vi "Name Strings to Version.vi"(9 "target name":string, 11 "robot model name (plugin name)":string) -> (0 "invalid inputs?":bool, 1 "FPGA target":T1, 3 "starter kit version":T2)   [LabVIEW 2017, in "NI_Robotics_Starter Kit Host_FPGA.lvclass"]
uses:
  <vilib>/robotics/Starter Kit/FPGA Host Interface/NI_Robotics_Starter Kit Host_FPGA.lvclass
  <vilib>/robotics/Starter Kit/Host Interface/Starter Kit Version.ctl
  <vilib>/robotics/Starter Kit/FPGA Host Interface/FPGA Target.ctl
  <vilib>/robotics/Starter Kit/Host Interface/NI_Robotics_Starter Kit Host.lvclass
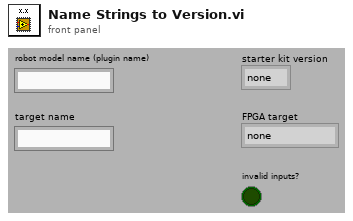
[diagram p1: front panel]
types:
  T1 = typedef "NI_Robotics_Starter Kit Host_FPGA.lvclass/FPGA Target.ctl" = enum16{"none", "sbRIO-9631", "sbRIO-9632", "sbRIO-9641", "sbRIO-9642"}
  T2 = typedef "NI_Robotics_Starter Kit Host.lvclass/Starter Kit Version.ctl" = enum16{"none", "1.0", "2.0"}
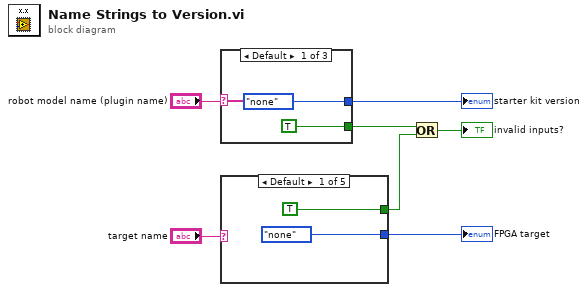
[diagram p0: block diagram]
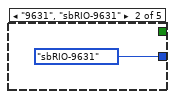
[diagram p2: hidden frame]
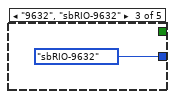
[diagram p3: hidden frame]
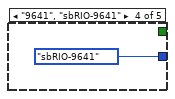
[diagram p4: hidden frame]
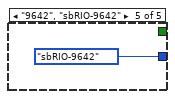
[diagram p5: hidden frame]
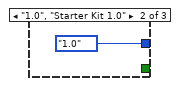
[diagram p6: hidden frame]
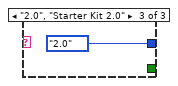
[diagram p7: hidden frame]
diagram:
  n1 = case shown="Default" "robot model name (plugin name)" {
    tunnel: [Starter_Kit_Version."none" ("starter kit version") Starter_Kit_Version."1.0" ("starter kit version") Starter_Kit_Version."2.0" ("starter kit version")] -> w5
    tunnel: [TRUE _ _] -> w3
    frame Default {
    }
    frame "1.0", "Starter Kit 1.0" {
    }
    frame "2.0", "Starter Kit 2.0" {
    }
  }
  "starter kit version" <- w5
  n2 = case shown="Default" "target name" {
    tunnel: [FPGA_Target."none" ("FPGA target") FPGA_Target."sbRIO-9631" ("FPGA target") FPGA_Target."sbRIO-9632" ("FPGA target") FPGA_Target."sbRIO-9641" ("FPGA target") FPGA_Target."sbRIO-9642" ("FPGA target")] -> w4
    tunnel: [TRUE _ _ _ _] -> w2
    frame Default {
    }
    frame "9631", "sbRIO-9631" {
    }
    frame "9632", "sbRIO-9632" {
    }
    frame "9641", "sbRIO-9641" {
    }
    frame "9642", "sbRIO-9642" {
    }
  }
  "FPGA target" <- w4
  n3 = Or(x=w3, y=w2) -> (x .or. y?=→"invalid inputs?":bool)
